vi "MS SQL_Count_RFID_STN90_V2.vi"(8 "error in (no error)":errorcluster, 11 "Ref in":T1={"MS SQL Connection"=refnum, "UDL File"=path "", "Time"="", "DCODE"="", "WIP+1"=0, "MC No?"=0, "POKAYOKE?"=FALSE, "Expected Result"="", "Result [Status]"="", "Clock"=0.0, "RFID"="", "WIP Queue"=refnum, "TS Parameter"={"ProfitCenterCode"="", "LineCode"="", "WorkOrderNumber"="", "Model"="", "Model_with_Prefix"="", "VendorCode"="", "SetParameterDateCode"="", "PokaYoke"=0, "Target"=1, "Live_DateCode"="", "CustomerPartNumber"="", "Hand"="", "Ent_Stamp"=timestamp(0 s since 1904-01-01), "STS_CD"=0.0}, "Data_Queue"=[], "RFID Serial No."=""} {"TS Parameter"."Target" min=1 max=100000; "TS Parameter"."PokaYoke" min=0 max=1}) -> (0 "error out":errorcluster, 1 "Count":i32 format="%02d", 2 "Count[s]":string, 3 "Ref OuT":T1={"MS SQL Connection"=refnum, "UDL File"=path "", "Time"="", "DCODE"="", "WIP+1"=0, "MC No?"=0, "POKAYOKE?"=FALSE, "Expected Result"="", "Result [Status]"="", "Clock"=0.0, "RFID"="", "WIP Queue"=refnum, "TS Parameter"={"ProfitCenterCode"="", "LineCode"="", "WorkOrderNumber"="", "Model"="", "Model_with_Prefix"="", "VendorCode"="", "SetParameterDateCode"="", "PokaYoke"=0, "Target"=1, "Live_DateCode"="", "CustomerPartNumber"="", "Hand"="", "Ent_Stamp"=timestamp(0 s since 1904-01-01), "STS_CD"=0.0}, "Data_Queue"=[], "RFID Serial No."=""} {"TS Parameter"."Target" min=1 max=100000; "TS Parameter"."PokaYoke" min=0 max=1})   [LabVIEW 2020]
uses:
  Controls/TD SQL.ctl
  <vilib>/addons/database/Connection.llb/Conn ObjectReference.ctl
  Controls/WIP_State.ctl
  Controls/TS_Parameter.ctl
  <vilib>/addons/database/NI_Database_API.lvlib
panel:
  out "resulting string":string
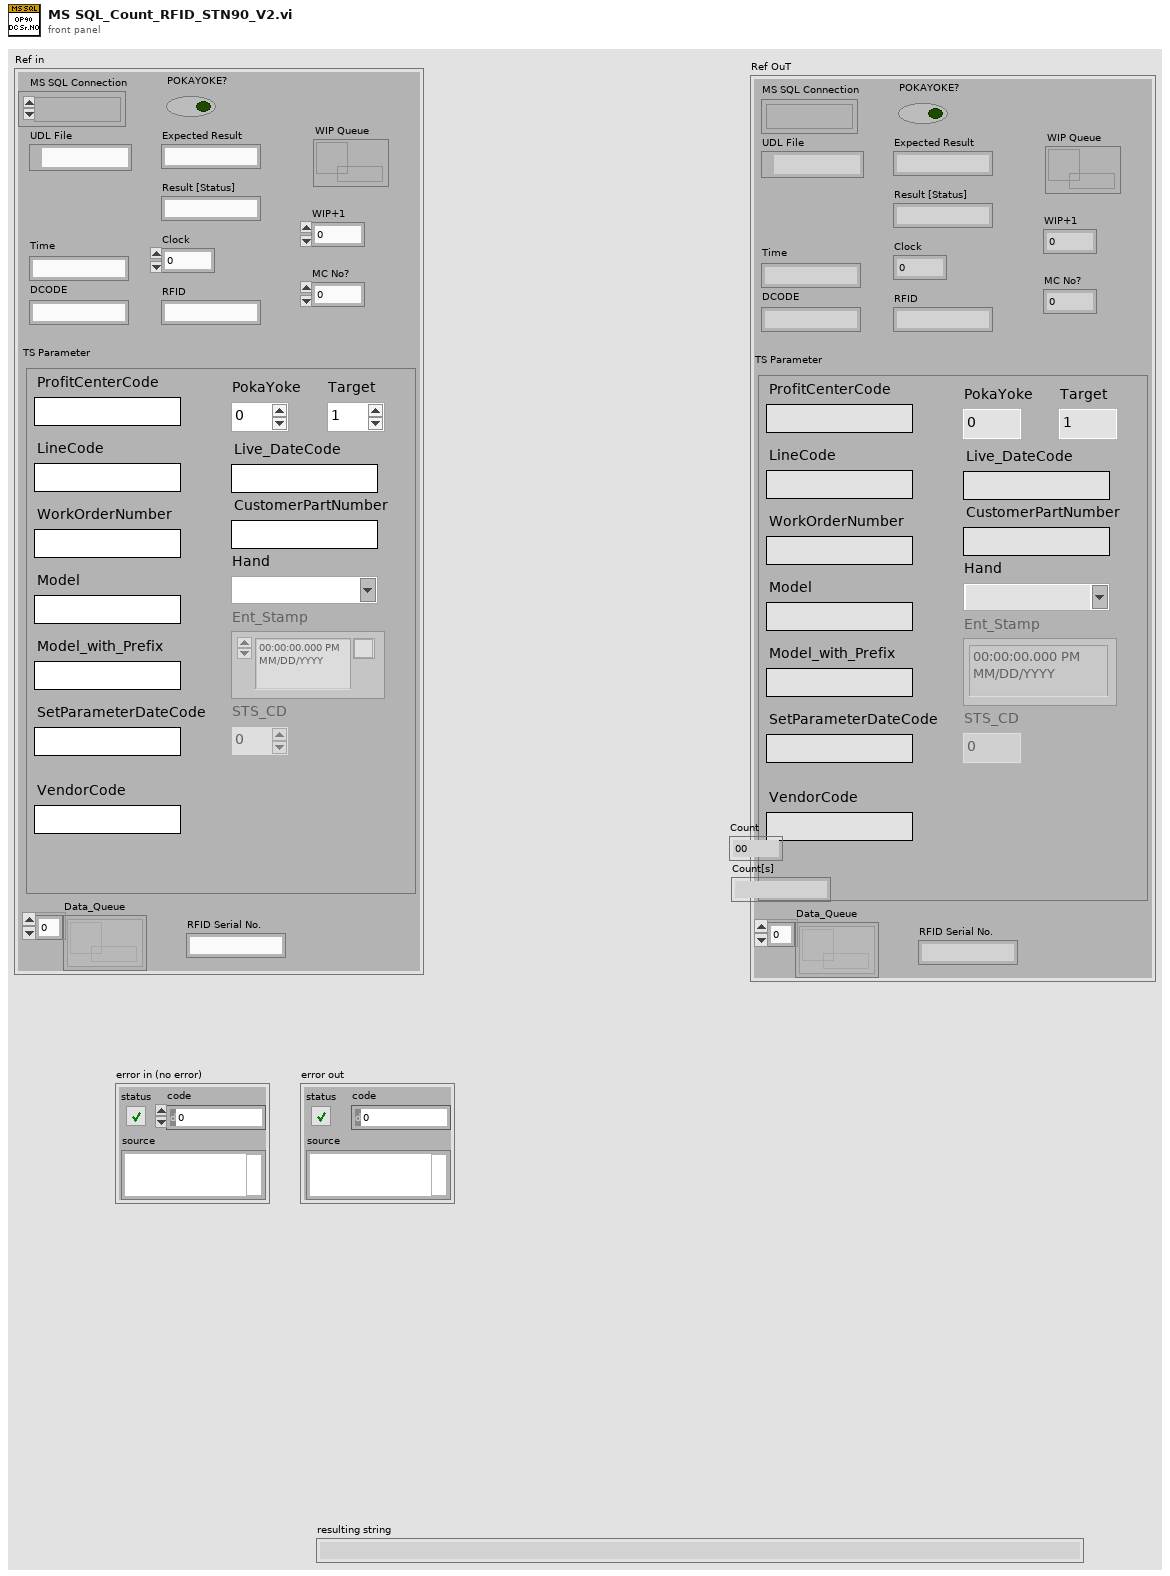
[diagram p1: front panel]
types:
  T1 = typedef "TD SQL.ctl" = cluster{"MS SQL Connection":T2, "UDL File":path, "Time":string, "DCODE":string, "WIP+1":i64, "MC No?":i32, "POKAYOKE?":bool, "Expected Result":string, "Result [Status]":string, "Clock":dbl, "RFID":string, "WIP Queue":refnum<queue>, "TS Parameter":T3, "Data_Queue":refnum<queue>[], "RFID Serial No.":string}
  T2 = typedef "NI_Database_API.lvlib/Conn ObjectReference.ctl" = refnum<k1>
  T3 = typedef "TS_Parameter.ctl" = cluster{"ProfitCenterCode":string, "LineCode":string, "WorkOrderNumber":string, "Model":string, "Model_with_Prefix":string, "VendorCode":string, "SetParameterDateCode":string, "PokaYoke":i32, "Target":i32, "Live_DateCode":string, "CustomerPartNumber":string, "Hand":string, "Ent_Stamp":timestamp, "STS_CD":dbl}
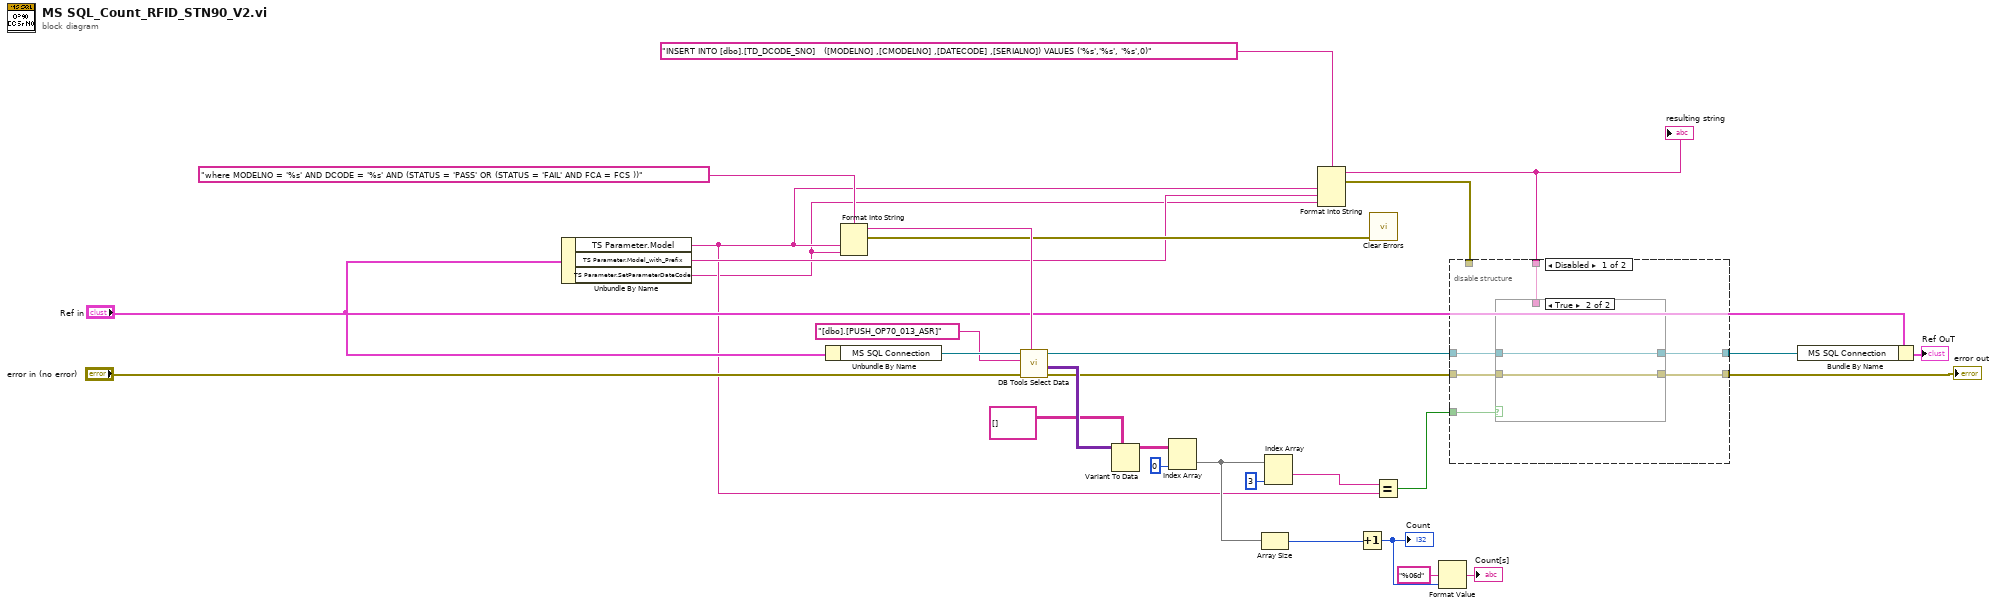
[diagram p0: block diagram]
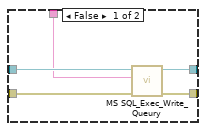
[diagram p2: hidden frame]
diagram:
  n1 = Unbundle By Name("Ref in") -> ("TS Parameter.Model"=w2:string, "TS Parameter.Model_with_Prefix"=w3:string, "TS Parameter.SetParameterDateCode"=w1:string)
  n2 = Unbundle By Name("Ref in") -> ("MS SQL Connection"=w28:T2)
  n3 = Format Into String(format string="where MODELNO = '%s' AND DCODE = '%s' AND (STATUS = 'PASS' OR (STATUS = 'FAIL' AND FCA = FCS ))", w2, w1) -> (resulting string=w23:string, error out=w19:errorcluster)  [unwired: 2 in]
  n4 = call <vilib>:"DB Tools Select Data.vi"("condition"=w23, "error in (no error)"="error in (no error)", "table"="[dbo].[PUSH_OP70_013_ASR]", "connection reference"=w28) -> ("error out"=w15:errorcluster, "data"=w22:variant[][], "connection reference out"=w17:T2)  [unwired: 2 in]
  n5 = Variant To Data(type=string[][] [] ("Data"), Variant=w22) -> (data=w18:string[][])  [unwired: 1 in, 1 out]
  n6 = Index Array(array=w18, index (col)=0 ("disabled index (col)")) -> (element=w7:string[])  [unwired: 1 in]
  n7 = Array Size(array=w7) -> (size(s)=w6:i32)
  n8 = Index Array(array=w7, index #2=3 ("index")) -> (element #1=w9:string)  [unwired: 1 in, 1 out]
  n9 = Format Into String(format string="INSERT INTO [dbo].[TD_DCODE_SNO]   ([MODELNO] ,[CMODELNO] ,[DATECODE] ,[SERIALNO]) VALUES ('%s','%s', '%s',0)" ("Query"), w2, w3, w1) -> (resulting string=w11:string, error out=w5:errorcluster)  [unwired: 2 in]
  "resulting string" <- w11
  n10 = Increment(x=w6) -> (x+1=w26:i32)
  "Count" <- w26
  n11 = call <vilib>:"Clear Errors.vi"("error in (no error)"=w19) -> ()  [unwired: 5 in, 2 out]
  n12 = Equal?(x=w9, y=w2) -> (x = y?=w13:bool)
  n13 = Format Value(format string="%06d", value (0)=w26) -> (output string=→"Count[s]":string)  [unwired: 1 in]
  n14 = disable-structure shown="Disabled" {
    disable-tunnel: w17 -> [w36 w45]
    disable-tunnel: [w35 w45] -> w16
    disable-tunnel: w15 -> [w34 w44]
    disable-tunnel: [w33 w44] -> w14
    disable-tunnel: w13 -> [w32 _]
    disable-tunnel: w11 -> [w31 _]
    disable-tunnel: w5 -> [_ _]
    frame Disabled {
      n15 = case shown="True" w32 {
        tunnel: w36 -> [w41 w43]
        tunnel: [w40 w43] -> w35
        tunnel: w34 -> [w39 w42]
        tunnel: [w38 w42] -> w33
        tunnel: w31 -> [w37 _]
        frame False {
          n16 = call "MS SQL_Exec_Write_Queury.vi"("error in (no error)"=w39, "Query"=w37, "Refnum in"=w41) -> ("error out"=w38:errorcluster, "Refnum out"=w40:T2)  [unwired: 7 in]
        }
        frame True {
        }
      }
    }
    frame Enabled {
    }
  }
  "error out" <- w14
  n17 = Bundle By Name(cluster="Ref in", "MS SQL Connection"=w16) -> (→"Ref OuT":T1)
